vi "grid-agent-simulator.vi"() -> ()   [LabVIEW 2021]
panel:
  out "ack":T1
  in  "change-mode-to":string(combo)
  in  "param":T2
  in  "base":cluster{"type":dbl, "mode":dbl, "sequence":dbl}
  in  "send-island":bool=TRUE
  in  "islanding-config":T3={"RA-ip"="127.0.0.1", "listen-port"=32101, "write-port"=32111}
  in  "send":bool=TRUE
  in  "main stop":bool
  in  "REQ":T4
  in  "daemon-config":T5={"resource-type"="battery", "agent-id"=12, "GA-ip"="192.168.1.1", "GA-port"=52020, "RA-ip"="127.0.0.1", "RA-port"=52001, "listenport-RA-side"=52011, "listenport-GA-side"=52021}
  # "ISLANDING COMMANDS"
  # "REQUESTS"
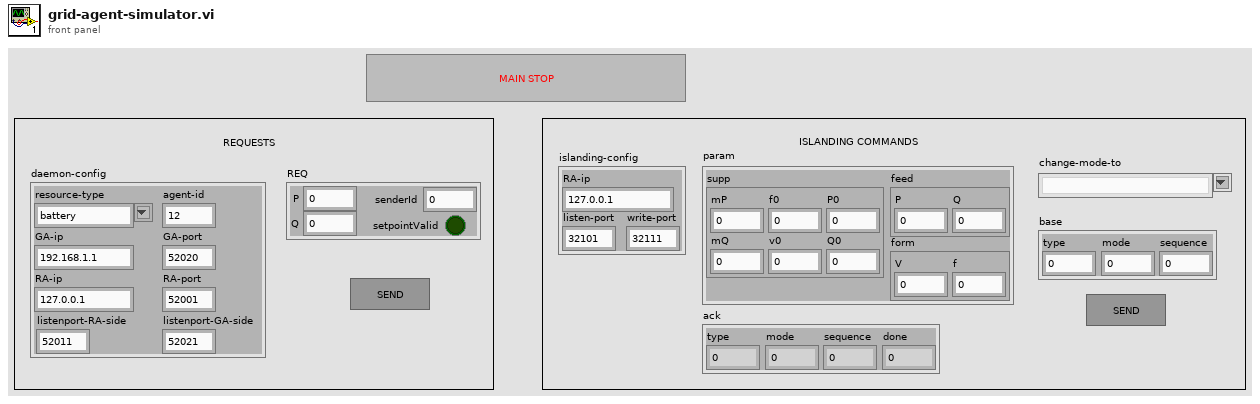
[diagram p1: front panel]
types:
  T1 = cluster{"type":dbl, "mode":dbl, "sequence":dbl, "done":dbl}
  T2 = cluster{"supp":cluster{"mP":dbl, "f0":dbl, "P0":dbl, "v0":dbl, "mQ":dbl, "Q0":dbl}, "form":cluster{"V":dbl, "f":dbl}, "feed":cluster{"P":dbl, "Q":dbl}}
  T3 = cluster{"RA-ip":string, "listen-port":u16, "write-port":u16}
  T4 = cluster{"P":dbl, "Q":dbl, "senderId":u32, "setpointValid":bool}
  T5 = cluster{"resource-type":string, "agent-id":u16, "GA-ip":string, "GA-port":u16, "RA-ip":string, "RA-port":u16, "listenport-RA-side":u16, "listenport-GA-side":u16}
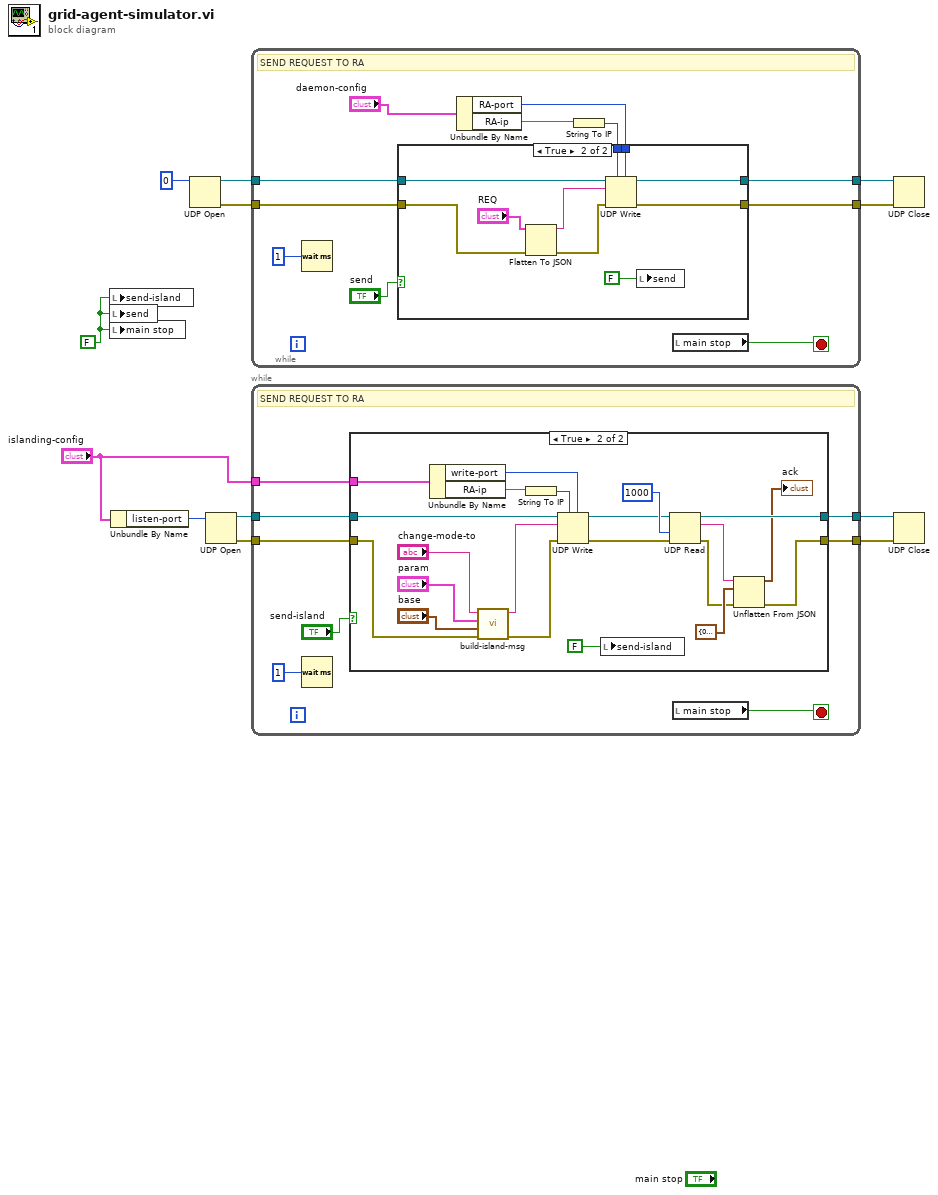
[diagram p0: block diagram]
diagram:
  w1 = FALSE ("main stop")
  n1 = local write "send-island"(w1) -> ()
  n2 = local write "send"(w1) -> ()
  n3 = local write "main stop"(w1) -> ()
  n4 = Unbundle By Name("islanding-config") -> ("listen-port"=w2:u16)
  n5 = UDP Open(11:u16 0 ("port")) -> (port=w10:refnum<k16>, 0:w9:errorcluster)  [unwired: 4 in, 1 out]
  n6 = UDP Open(11:w2) -> (port=w5:refnum<k16>, 0:w4:errorcluster)  [unwired: 4 in, 1 out]
  n7 = while {
    tunnel: w10 -> [w21]
    tunnel: w9 -> [w22]
    tunnel: [w19] -> w12
    tunnel: [w18] -> w11
    stop <- w23 stop-if-true
    # "SEND REQUEST TO RA"
    n8 = Wait (ms)(milliseconds to wait=u32 1) -> ()  [unwired: 1 out]
    n9 = Unbundle By Name("daemon-config") -> ("RA-port"=w15:u16, "RA-ip"=w17:string)
    n10 = String To IP(1:w17) -> (0:w16:u32)
    n11 = case shown="True" "send" {
      tunnel: w22 -> [w24 w34]
      tunnel: w21 -> [w25 w33]
      tunnel: [w25 w30] -> w19
      tunnel: [w24 w29] -> w18
      tunnel: w16 -> [_ w28]
      tunnel: w15 -> [_ w27]
      frame False {
      }
      frame True {
        n12 = Flatten To JSON(anything="REQ", error in (no error)=w34) -> (JSON string=w26:string, 11:w32:errorcluster)  [unwired: 1 in]
        n13 = UDP Write(address=w28, port or service name=w27, connection ID=w33, data in=w26, 8:w32) -> (error out=w29:errorcluster, 3:w30:refnum<k16>)  [unwired: 1 in]
        n14 = local write "send"(FALSE) -> ()
      }
    }
    n15 = local read "main stop"() -> (w23:bool)
  }
  n16 = while {
    tunnel: w5 -> [w41]
    tunnel: w4 -> [w42]
    tunnel: [w39] -> w7
    tunnel: [w38] -> w6
    tunnel: "islanding-config" -> [w36]
    stop <- w43 stop-if-true
    # "SEND REQUEST TO RA"
    n17 = Wait (ms)(milliseconds to wait=u32 1) -> ()  [unwired: 1 out]
    n18 = case shown="True" "send-island" {
      tunnel: w42 -> [w44 w62]
      tunnel: w41 -> [w45 w66]
      tunnel: [w45 w52] -> w39
      tunnel: [w44 w46] -> w38
      tunnel: w36 -> [_ w57]
      frame False {
      }
      frame True {
        n19 = Unbundle By Name(w57) -> ("write-port"=w55:u16, "RA-ip"=w58:string)
        n20 = call "build-island-msg.vi"("error (in)"=w62, "base"="base", "param"="param", "change-mode-to"="change-mode-to") -> ("error (out)"=w63:errorcluster, "JSON string"=w64:string)  [unwired: 2 in]
        n21 = String To IP(1:w58) -> (0:w56:u32)
        n22 = UDP Write(address=w56, port or service name=w55, connection ID=w66, data in=w64, 8:w63) -> (error out=w51:errorcluster, 3:w53:refnum<k16>)  [unwired: 1 in]
        n23 = local write "send-island"(FALSE) -> ()
        n24 = UDP Read(connection ID=w53, timeout ms (25000)=1000, 8:w51) -> (data out=w48:string, error out=w47:errorcluster, 3:w52:refnum<k16>)  [unwired: 3 out]
        n25 = Unflatten From JSON(JSON string=w48, type and defaults=T1 {"type"=0.0, "mode"=0.0, "sequence"=0.0, "done"=0.0} ("ack"), error in (no error)=w47) -> (value=→"ack":T1, error out=w46:errorcluster)  [unwired: 4 in]
      }
    }
    n26 = local read "main stop"() -> (w43:bool)
  }
  n27 = UDP Close(connection ID=w12, 8:w11) -> ()  [unwired: 2 out]
  n28 = UDP Close(connection ID=w7, 8:w6) -> ()  [unwired: 2 out]
